vi "Timestamp s4ics.vi"(10 "subsystem":string) -> (2 "system timestamp":string)   [LabVIEW 2018]
panel:
  # "ISO 8601:\nSeptember 27, 2022 at 6 p.m. is represented as 2022-09-27 18:00:00.000."
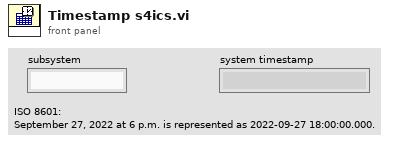
[diagram p1: front panel]
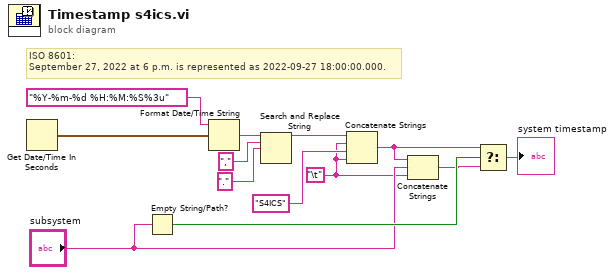
[diagram p0: block diagram]
diagram:
  w1 = "\t"
  # "ISO 8601:\nSeptember 27, 2022 at 6 p.m. is represented as 2022-09-27 18:00:00.000."
  n1 = Get Date/Time In Seconds() -> (seconds since 1Jan1904=w9:timestamp)
  n2 = Empty String/Path?(string/path="subsystem") -> (empty?=w8:bool)
  n3 = Format Date/Time String(time format string (%c)="%Y-%m-%d %H:%M:%S%3u", seconds (now)=w9) -> (date/time string=w12:string)  [unwired: 1 in]
  n4 = Search and Replace String(input string=w12, search string=",", replace string=".") -> (result string=w2:string)  [unwired: 5 in, 3 out]
  n5 = Concatenate Strings(w2, w1, "S4ICS" ("system"), w1) -> (w5:string)
  n6 = Concatenate Strings(w5, "subsystem", w1) -> (w3:string)
  n7 = Select(t=w5, s=w8, f=w3) -> (s? t:f=→"system timestamp":string)
